vi "Get Keep Clean Time.vi"(8 "error in (no error)":errorcluster, 11 "KeepCleanTime":sgl) -> (0 "error out":errorcluster, 2 "function return":u32, 3 "KeepCleanTime out":sgl)   [LabVIEW 2014, in "atmcd32d.lvlib"]
doc: "unsigned int WINAPI GetKeepCleanTime(float * KeepCleanTime);"
uses:
  atmcd32d.lvlib
  atmcd32d.dll
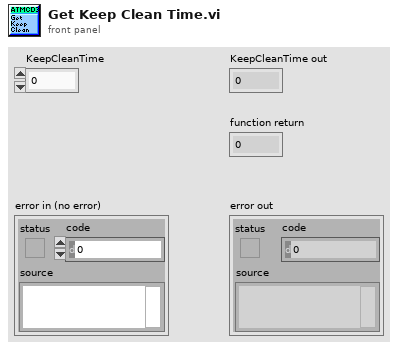
[diagram p1: front panel]
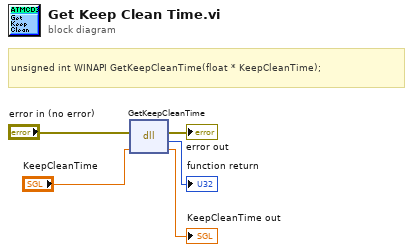
[diagram p0: block diagram]
diagram:
  # "unsigned int WINAPI GetKeepCleanTime(float * KeepCleanTime);"
  n1 = dll-call lib="C:/Users/Bakir/Documents/Lambda2-Testing/lib/Andorlib/atmcd32d.*" fn="GetKeepCleanTime"(error in="error in (no error)", "KeepCleanTime"="KeepCleanTime") -> (error out=→"error out":errorcluster, →"function return":u32, "KeepCleanTime"=→"KeepCleanTime out":sgl)  [unwired: 2 in, 1 out]
